vi "general data plot.vi"() -> ()   [LabVIEW 2021]
panel:
  in  "length":i32
  in  "start":i32
  out "min value":dbl
  out "max value":dbl=7.0
  in  "Data channel":u16(ring) items=["magitude", "phase", "i", "q"]
  in  "y bin":i32=100
  in  "x bin":i32=100
  in  "Tab Control":T1(tab)
  out "Curves":cluster{dbl[], dbl[]}[](graph)=[{[10.0, 20.0, 30.0, 40.0, 50.0, 60.0, 70.0, 80.0, 90.0, 100.0, 110.0, 120.0, 130.0, 140.0, 150.0, 160.0, 170.0, 180.0, 190.0, 200.0, 210.0, 220.0, 230.0, 240.0, 250.0, 260.0, 270.0, 280.0, 290.0, 300.0, 310.0, 320.0, 330.0, 340.0, 350.0, 360.0, 370.0, 380.0, 390.0, 400.0, 410.0, 420.0, 430.0, 440.0, 450.0, 460.0, 470.0, 480.0, 490.0, 500.0, 510.0, 520.0, 530.0, 540.0, 550.0, 560.0, 570.0, 580.0, 590.0, 600.0, 610.0, 620.0, 630.0, 640.0, 650.0, 660.0, 670.0, 680.0, 690.0, 700.0, 710.0, 720.0, 730.0, 740.0, 750.0, 760.0, 770.0, 780.0, 790.0, 800.0, 810.0, 820.0, 830.0, 840.0, 850.0, 860.0, 870.0, 880.0, 890.0, 900.0, 910.0, 920.0, 930.0, 940.0, 950.0, 960.0, 970.0, 980.0, 990.0, 1000.0, 1010.0, 1020.0, 1030.0, 1040.0, 1050.0, 1060.0, 1070.0, 1080.0, 1090.0, 1100.0, 1110.0, 1120.0, 1130.0, 1140.0, 1150.0, 1160.0, 1170.0, 1180.0, 1190.0, 1200.0, 1210.0, 1220.0, 1230.0, 1240.0, 1250.0, 1260.0, 1270.0, 1280.0, 1290.0, 1300.0, 1310.0, 1320.0, 1330.0, 1340.0, 1350.0, 1360.0, 1370.0, 1380.0, 1390.0, 1400.0, 1410.0, 1420.0, 1430.0, 1440.0, 1450.0, 1460.0, 1470.0, 1480.0, 1490.0, 1500.0, 1510.0, 1520.0, 1530.0, 1540.0, 1550.0, 1560.0, 1570.0, 1580.0, 1590.0, 1600.0, 1610.0, 1620.0, 1630.0, 1640.0, 1650.0, 1660.0, 1670.0, 1680.0, 1690.0, 1700.0, 1710.0, 1720.0, 1730.0, 1740.0, 1750.0, 1760.0, 1770.0, 1780.0, 1790.0, 1800.0, 1810.0, 1820.0, 1830.0, 1840.0, 1850.0, 1860.0, 1870.0, 1880.0, 1890.0, 1900.0, 1910.0, 1920.0, 1930.0, 1940.0, 1950.0, 1960.0, 1970.0, 1980.0, 1990.0, 2000.0, 2010.0, 2020.0, 2030.0, 2040.0, 2050.0, 2060.0, 2070.0, 2080.0, 2090.0, 2100.0, 2110.0, 2120.0, 2130.0, 2140.0, 2150.0, 2160.0, 2170.0, 2180.0, 2190.0, 2200.0, 2210.0, 2220.0, 2230.0, 2240.0, 2250.0, 2260.0, 2270.0, 2280.0, 2290.0, 2300.0, 2310.0, 2320.0, 2330.0, 2340.0, 2350.0, 2360.0, 2370.0, 2380.0, 2390.0, 2400.0, 2410.0, 2420.0, 2430.0, 2440.0, 2450.0, 2460.0, 2470.0, 2480.0, 2490.0, 2500.0, 2510.0, 2520.0, 2530.0, 2540.0, 2550.0, 2560.0, 2570.0, 2580.0, 2590.0, 2600.0, 2610.0, 2620.0, 2630.0, 2640.0, 2650.0, 2660.0, 2670.0, 2680.0, 2690.0, 2700.0, 2710.0, 2720.0, 2730.0, 2740.0, 2750.0, 2760.0, 2770.0, 2780.0, 2790.0, 2800.0, 2810.0, 2820.0, 2830.0, 2840.0, 2850.0, 2860.0, 2870.0, 2880.0, 2890.0, 2900.0, 2910.0, 2920.0, 2930.0, 2940.0, 2950.0, 2960.0, 2970.0, 2980.0, 2990.0], [0.00013367658539209515, 0.00012903053720947355, 0.00016939388297032565, 0.00011944288416998461, 0.00013280082202982157, 0.0001668874901952222, 0.0001486373512307182, 0.00016734786913730204, 0.00013047773973084986, 0.00011366923718014732, 0.00015346240252256393, 0.00014055744395591319, 0.00010855273285415024, 0.00014807406114414334, 9.691778541309759e-05, 0.0001037847250699997, 0.00015512084064539522, 0.00012899791181553155, 0.00010304365423507988, 0.00010984897380694747, 9.950714593287557e-05, 0.00012845687160734087, 9.946813952410594e-05, 0.00013071915600448847, 0.00010318124259356409, 7.330832886509597e-05, 9.540999599266797e-05, 8.451899338979274e-05, 0.00011770859418902546, 0.00010144653788302094, 0.00010661190026439726, 9.66657607932575e-05, 8.824256656225771e-05, 0.00011671280662994832, 0.0001153357297880575, 0.00012023511953884736, 0.00011908653686987236, 7.182291301432997e-05, 9.330980537924916e-05, 0.00012978495215065777, 0.00010747888882178813, 0.0001609536848263815, 0.00012383898138068616, 0.00012734768097288907, 0.00013171030150260776, 0.00016544826212339103, 0.00011794555030064657, 0.0001209946713061072, 0.00013883289648219943, 0.00011528369941515848, 0.00011119921691715717, 0.0001268050546059385, 0.0001389453827869147, 0.0001333432155661285, 0.0001442368666175753, 0.00013873385614715517, 0.00015191496640909463, 0.0001383038325002417, 0.00016562323435209692, 0.0001503702369518578, 0.00018218863988295197, 0.00015577522572129965, 0.00013113849854562432, 0.0001594854547875002, 0.0001855860318755731, 0.00019237845845054835, 0.00016393935948144644, 0.00012862142466474324, 0.00020546221639961004, 0.00017347501125186682, 0.00016879066242836416, 0.00018185762746725231, 0.00021324920817278326, 0.0001671143400017172, 0.00017139053670689464, 0.00019904927466996014, 0.00020881103409919888, 0.0001565761340316385, 0.00017052458133548498, 0.00014252751134335995, 0.00014181881851982325, 0.0001779100566636771, 0.00014105757873039693, 0.00018711318261921406, 0.00016824345220811665, 0.00015031950897537172, 0.0002022298431256786, 0.0001394925347995013, 0.00019517798500601202, 0.00016337772831320763, 0.00016140898515004665, 0.00015929783694446087, 0.00019489617261569947, 0.0001588258455740288, 0.00019977384363301098, 0.00012394576333463192, 0.00013413015403784811, 0.00019717543909791857, 0.00018152548000216484, 0.0001585373393027112, 0.00018475871183909476, 0.0001751347881508991, 0.00018880412972066551, 0.00014899946108926088, 0.00014845613623037934, 0.0001744086475810036, 0.0001450015843147412, 0.00016606866847723722, 0.00014761251804884523, 0.00012996570148970932, 0.000138217699714005, 0.00010744725295808166, 0.00014905130956321955, 0.00011166420881636441, 0.0001041400246322155, 0.0001146040522144176, 7.99687477410771e-05, 7.002366328379139e-05, 0.00017626908083911985, 0.00010617077350616455, 9.990988473873585e-05, 6.87278006807901e-05, 8.242046169470996e-05, 8.596655243309215e-05, 0.00014996137178968638, 8.169219654519111e-05, 0.0001243894948856905, 0.00014897635264787823, 0.0001250183704541996, 0.000117989067803137, 0.00012694876932073385, 0.00015508588694501668, 9.217203478328884e-05, 9.355860674986616e-05, 0.00010396670404588804, 9.367567690787837e-05, 8.306658128276467e-05, 9.193496953230351e-05, 9.813846554607153e-05, 0.00011742529750335962, 6.46550688543357e-05, 0.00013626340660266578, 0.00012126795627409592, 0.0001021269999910146, 0.0001304978650296107, 9.543891792418435e-05, 0.00013903676881454885, 0.00011544466542545706, 0.00013386114733293653, 0.0001186947338283062, 0.00010264376760460436, 0.00018659705528989434, 0.00010800208838190883, 0.00014367169933393598, 0.00011846152483485639, 7.385665958281606e-05, 0.0001364771305816248, 0.00011073373752878979, 0.00010194589413003996, 0.00014044092677067965, 8.428201545029879e-05, 0.00012676689948420972, 0.0001338515430688858, 0.00010269197809975594, 0.00023462837270926684, 0.00013209556345827878, 0.00010225973528577015, 0.000106790590507444, 0.00017195282271131873, 9.286184649681672e-05, 0.00012535882706288248, 0.000116468254418578, 9.88127212622203e-05, 0.00010617675434332341, 7.647919119335711e-05, 9.201795910485089e-05, 0.00010408402886241674, 9.458380372961983e-05, 0.0001077998531400226, 0.00011431352322688326, 0.00010332229430787265, 0.00011219579027965665, 0.0001334812113782391, 0.00014534480578731745, 0.00011573600932024419, 6.758727977285162e-05, 0.0001744368055369705, 0.00016830879030749202, 0.00017424295947421342, 0.00016627485456410795, 0.00012254131434019655, 9.647793922340497e-05, 7.145500421756878e-05, 0.0001961914385901764, 7.151101453928277e-05, 0.00012814125511795282, 9.786655573407188e-05, 0.00010398540325695649, 0.00010584685514913872, 0.00015125608479138464, 0.00012826750753447413, 5.975702151772566e-05, 0.00013089587446302176, 0.00012053469254169613, 0.00015860950225032866, 6.76583731546998e-05, 8.026184514164925e-05, 0.00013365043560042977, 6.834783562226221e-05, 5.882106052013114e-05, 7.937144255265594e-05, 8.463740959996358e-05, 8.238392183557153e-05, 9.121077164309099e-05, 0.00012566435907501727, 5.283867722027935e-05, 0.0001325753692071885, 0.0001193397692986764, 0.00011944347352255136, 0.00010491804277990013, 7.044597441563383e-05, 7.60913681006059e-05, 9.172792488243431e-05, 0.00011764467490138486, 5.072560816188343e-05, 5.034092100686394e-05, 9.650958236306906e-05, 0.00011145589814987034, 8.698977762833238e-05, 0.00013060042692814022, 7.508155249524862e-05, 4.039569466840476e-05, 0.00012688440619967878, 8.248807716881856e-05, 0.0001391138503095135, 0.00011811658623628318, 0.0001329777151113376, 0.0001297980488743633, 0.00011801200162153691, 7.027927495073527e-05, 8.611835073679686e-05, 8.903844718588516e-05, 5.4920932598179206e-05, 0.00010779354488477111, 8.671233081258833e-05, 7.775093399686739e-05, 0.00012373703066259623, 0.00010819485760293901, 0.00010179568198509514, 8.725826046429574e-05, 9.490929369349033e-05, 0.0001120992237702012, 0.0001260258286492899, 6.4598280005157e-05, 0.00011466383148217574, 0.00014919301611371338, 9.42891783779487e-05, 9.435992251383141e-05, 0.0001149402596638538, 8.329037518706173e-05, 0.00010850686521735042, 0.0001287714985664934, 0.00013188911543693393, 0.00011211052333237603, 0.0001296363479923457, 0.0001389684621244669, 0.0001123499168897979, 9.72454363363795e-05, 9.088624938158318e-05, 9.20691090868786e-05, 8.7498570792377e-05, 0.0001258686388609931, 0.00013619156379718333, 8.844014519127086e-05, 0.00012676880578510463, 8.672325202496722e-05, 0.00013719592243433, 0.000103384954854846, 7.913039007689804e-05, 7.551917224191129e-05, 7.993963663466275e-05, 0.0001514438772574067, 0.000121453391329851, 0.00014526258746627718, 0.00011735747830243781, 9.341667464468628e-05, 8.561307186027989e-05, 0.00013149157166481018, 0.00010279854177497327, 9.32314433157444e-05, 0.0001331145758740604, 8.938983228290454e-05, 0.00013474171282723546, 0.0001676843239692971, 8.821023220662028e-05, 0.00011201468441868201, 0.0001366356445942074, 0.00013054072041995823, 0.00016769583453424275]}]
  out "distribution":dbl[][](graph)
  in  "Dist Marker Values":cluster{"Numeric":dbl, "Color Box":u32}[](array[cluster])=[{"Numeric"=0.0, "Color Box"=16448250}, {"Numeric"=10.0, "Color Box"=16711686}, {"Numeric"=14.0, "Color Box"=16860}]
  out "Y Cut":T2(graph)
  out "Intensity plot":dbl[][](graph)
  in  "Intensity Marker Values":cluster{"Numeric":dbl, "Color Box":u32}[](array[cluster])
  out "error out":errorcluster
  out "Axis array":dbl[](array[numeric])
  in  "Y Label":string(combo)="Mag"
  in  "X Label":string(combo)="Length ns"
  in  "y col":i32=1
  in  "x col":i32
  in  "Plot Type":string(combo)="iq vs x"
  in  "Plot":bool
  out "Status":string(combo)="Idle"
  in  "Stop":bool
  in  "update":bool
  in  "Data files":i32[](listbox)=[168]
  in  "Main folder path":path=path "C:/Users/dvh-collab-user/Desktop/20230313 Robert sample"
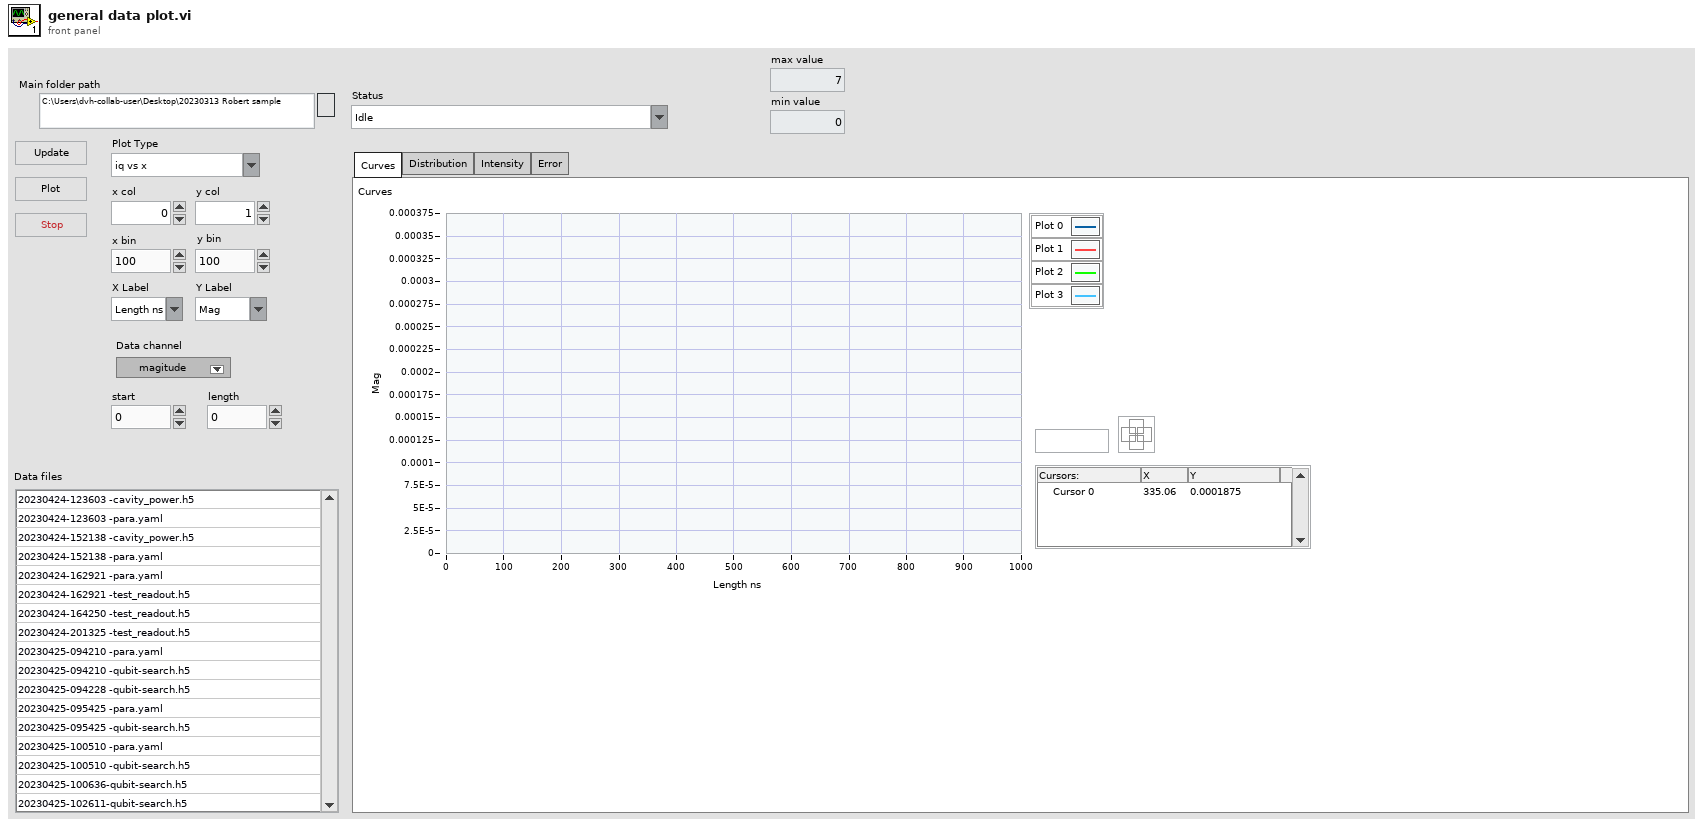
[diagram p1: front panel]
types:
  T1 = enum32{"Curves", "Distribution", "Intensity", "Error"}
  T2 = cluster{"Axis array":dbl[], "Intensity plot":dbl[]}
  T3 = cluster{" x min":dbl, "x step":dbl, "y min":dbl, "y step":dbl}
  T4 = cluster{"xname":string, "x_offset":dbl, "x_step":dbl, "yname":string, "y_offset":dbl, "y_step":dbl}
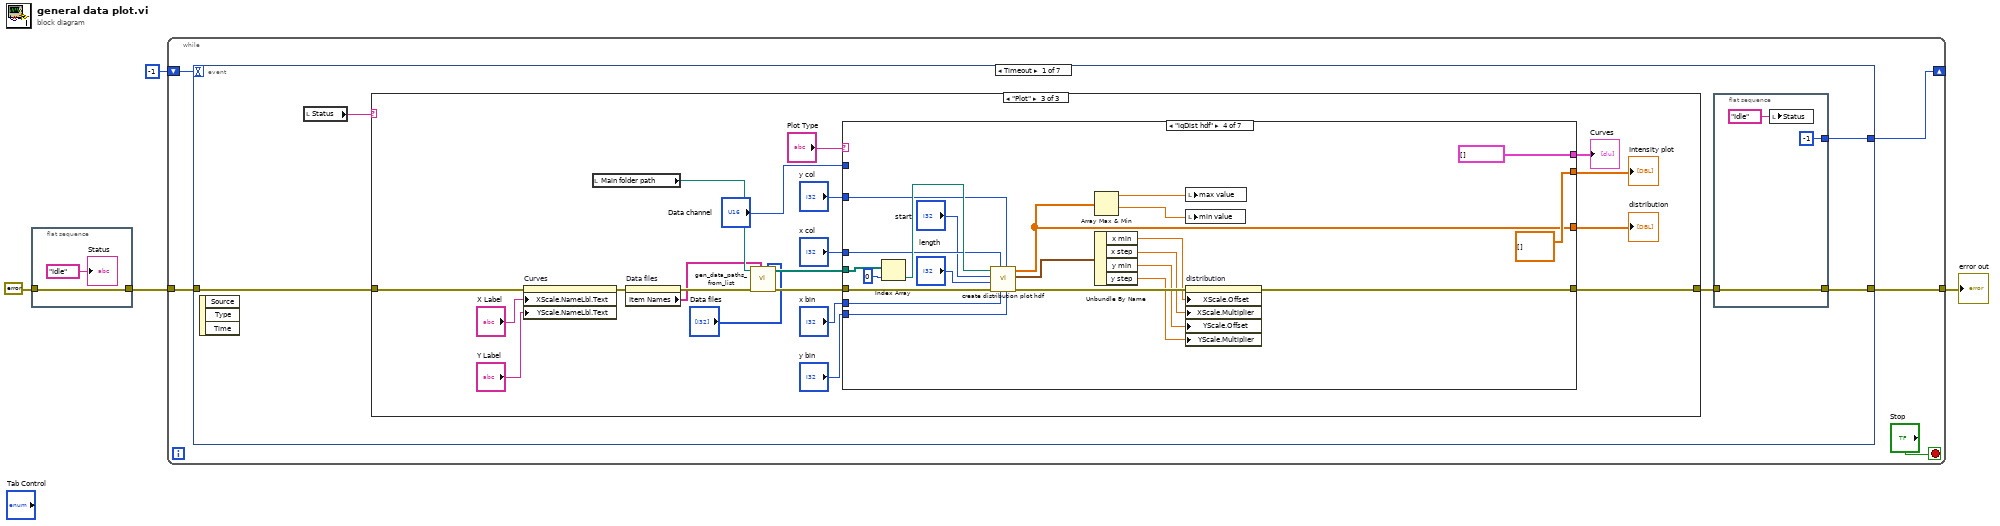
[diagram p0: block diagram]
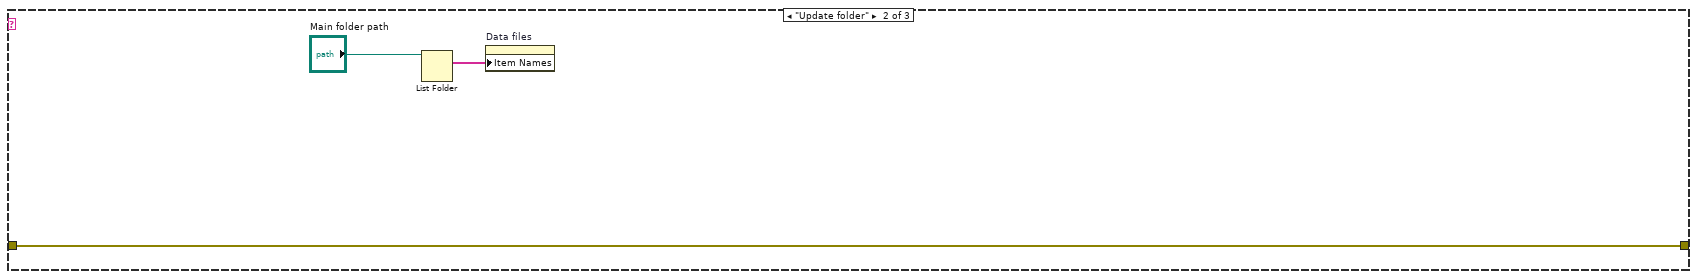
[diagram p3: hidden frame]
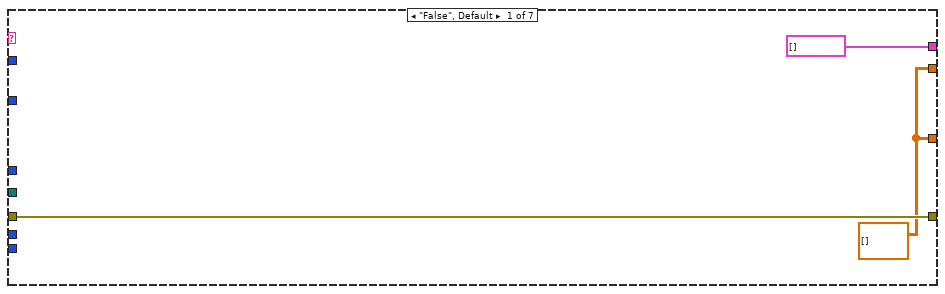
[diagram p4: hidden frame]
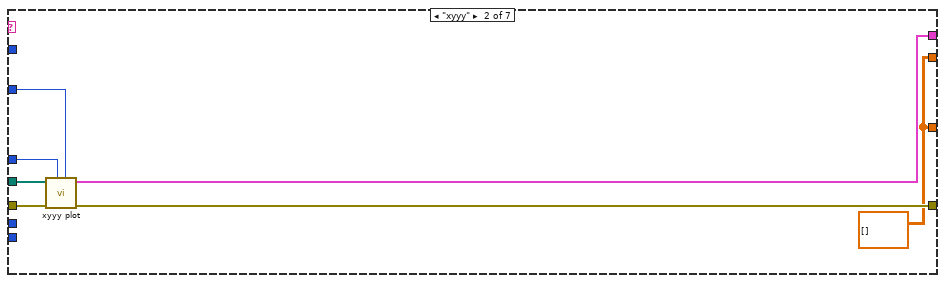
[diagram p5: hidden frame]
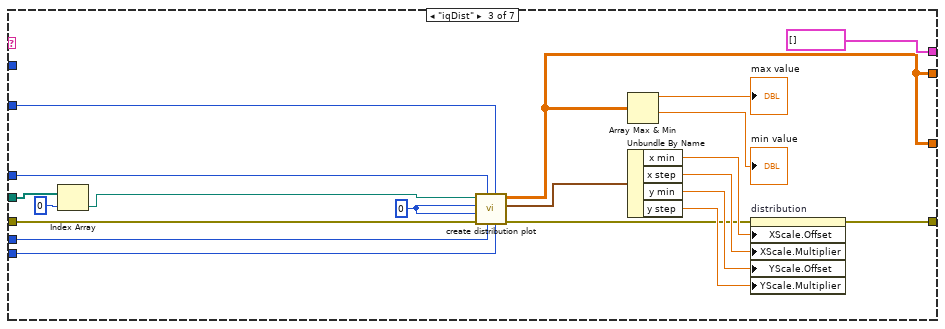
[diagram p6: hidden frame]
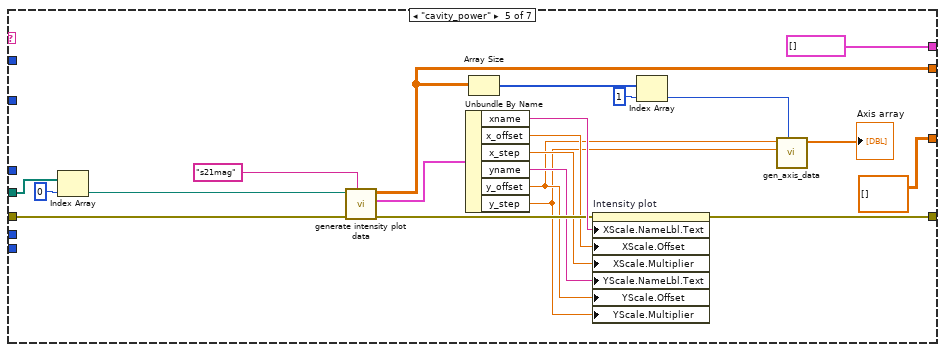
[diagram p7: hidden frame]
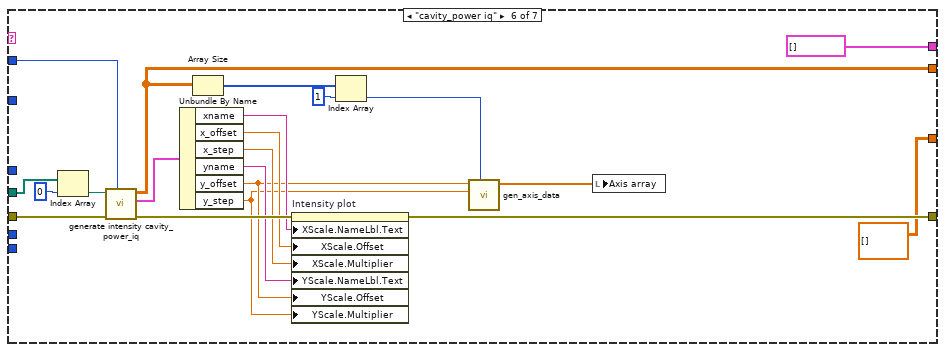
[diagram p8: hidden frame]
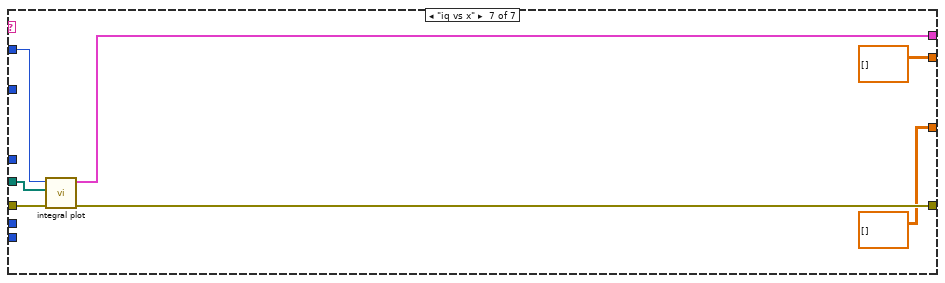
[diagram p9: hidden frame]
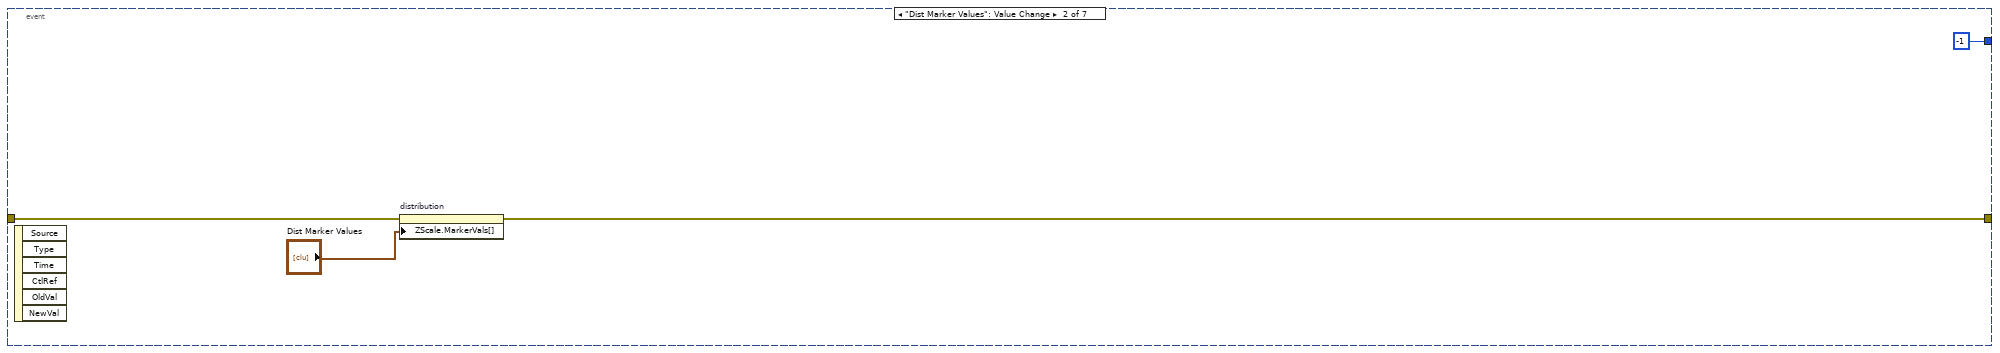
[diagram p10: hidden frame]
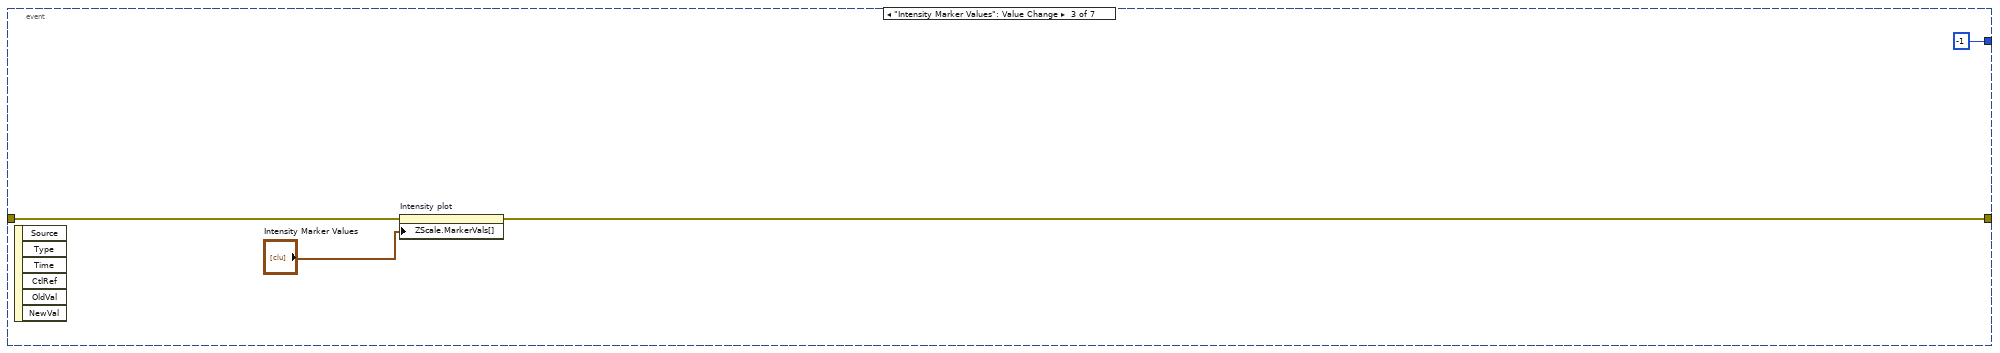
[diagram p11: hidden frame]
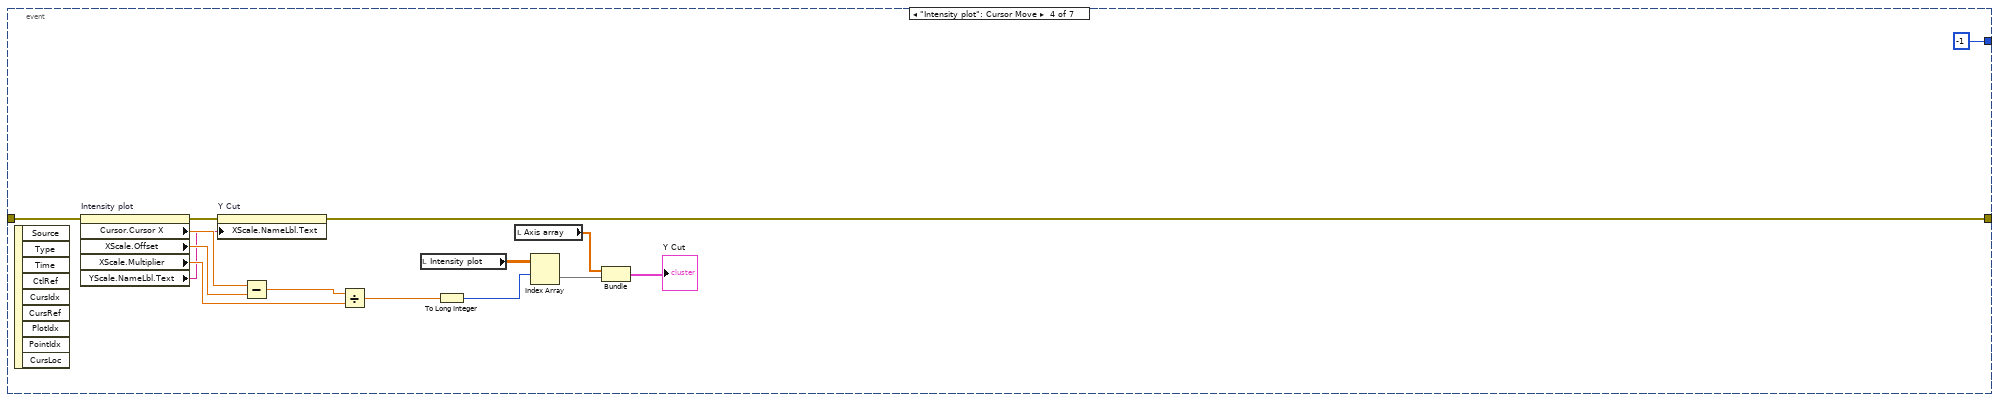
[diagram p12: hidden frame]
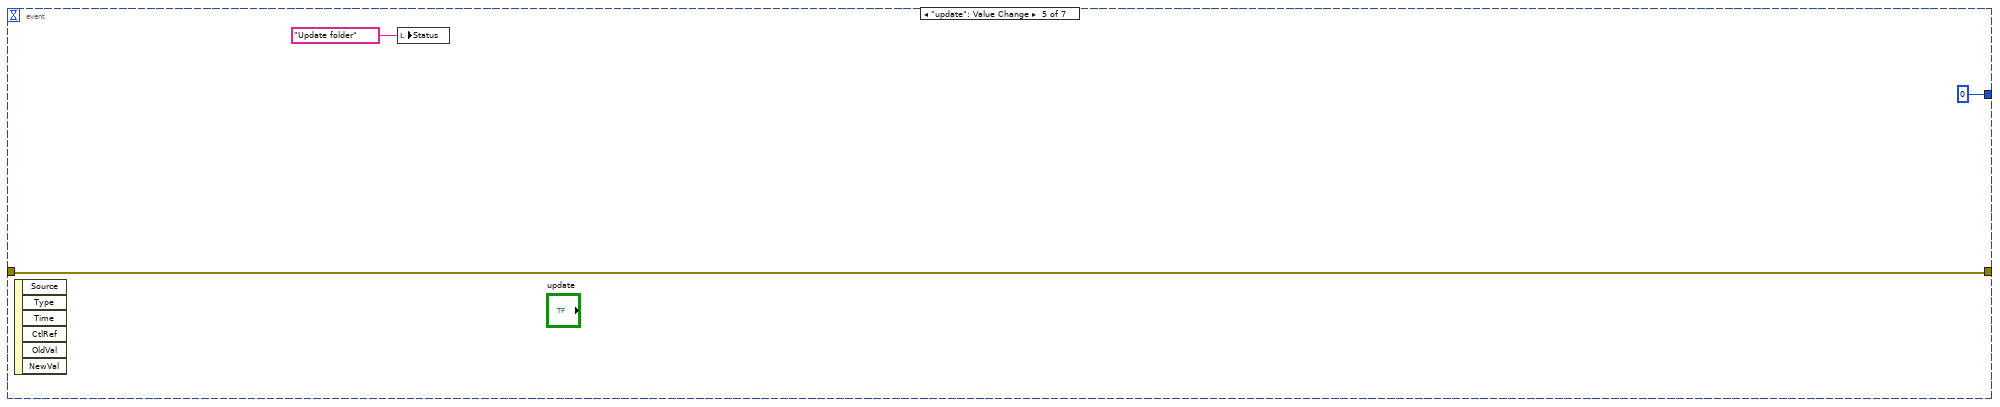
[diagram p13: hidden frame]
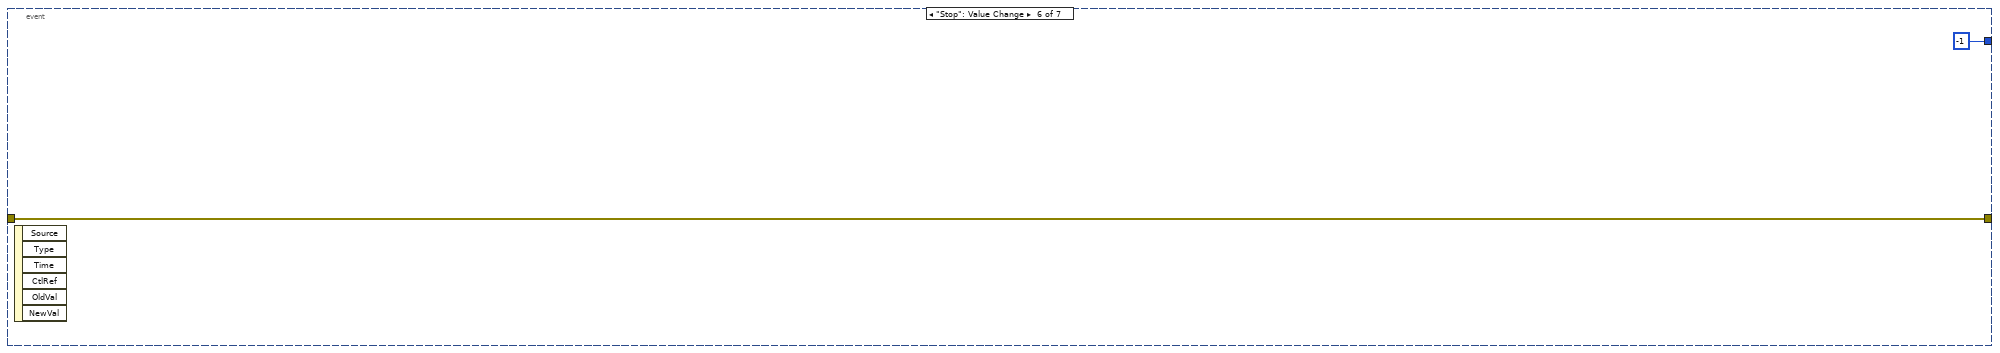
[diagram p14: hidden frame]
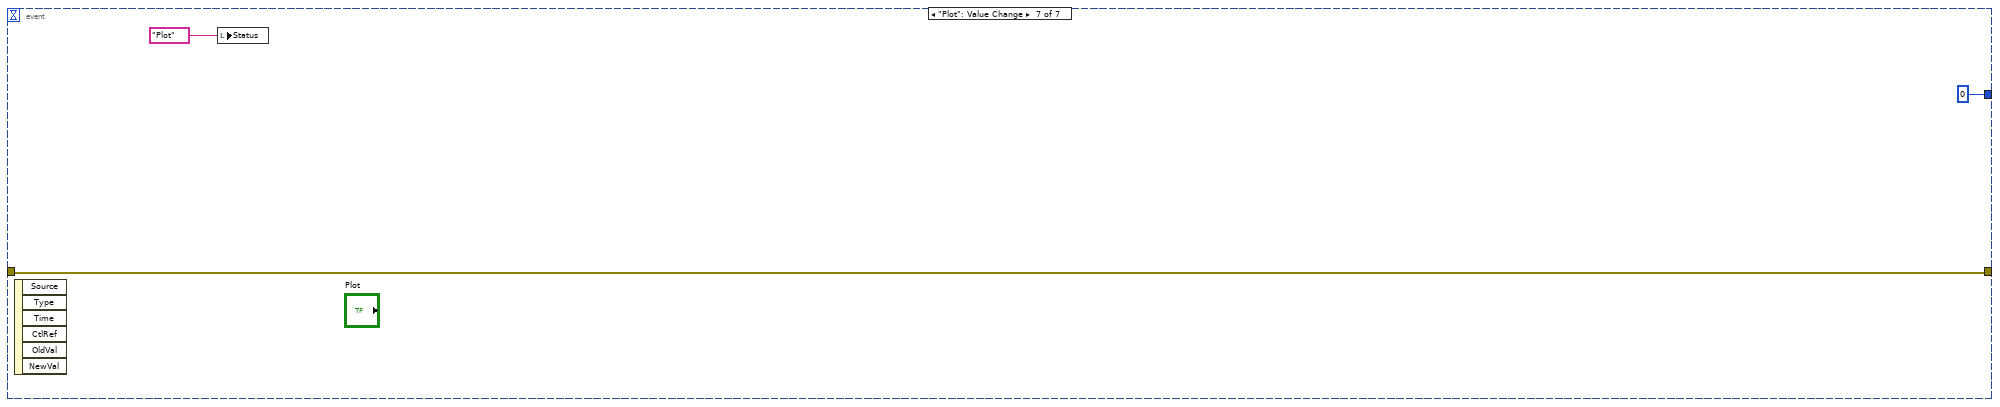
[diagram p15: hidden frame]
diagram:
  n1 = flat-sequence {
    tunnel: [w5] -> w2
    tunnel: errorcluster {"status"=FALSE, "code"=0, "source"=""} ("error in") -> [w5]
    frame #0 {
      "Status" <- "Idle" ("Status")
    }
  }
  n2 = while {
    shift-right: [w10] -> _
    shift-left: -1 -> [w11]
    tunnel: w2 -> [w9]
    tunnel: [w8] -> w1
    stop <- "Stop" stop-if-true
    n3 = event shown="[0] Timeout" {
      selector: _ -> [_ _ _ _ _ _ _]
      dyn-events: _ -> [_ _ _ _ _ _ _]
      timeout: w11 -> [_ _ _ _ _ _ _]
      tunnel: [w12 -1 -1 -1 0 -1 0] -> w10
      tunnel: w9 -> [w15 w147 w150 w167 w168 w172 w175]
      tunnel: [w13 w145 w152 w154 w168 w172 w175] -> w8
      event Timeout {
        n4 = event-data() -> ()  [unwired: 1 in, 3 out]
        n5 = local read "Status"() -> (w16:string)
        n6 = case shown="\"Plot\"" w16 {
          tunnel: [w20 w21 w39] -> w14
          tunnel: w15 -> [w20 w21 w32]
          frame "False", Default {
          }
          frame "Update folder" {
            n7 = List Folder(path="Main folder path") -> (filenames=w23:string[])  [unwired: 3 in, 3 out]
            n8 = property on="Data files" class="LstBox (strict)"("Item Names"=w23) -> ()  [unwired: 2 in, 2 out]
          }
          frame "Plot" {
            n9 = property on="Curves" class="XYGraph (strict)"(error in=w32, "XScale.NameLbl.Text"="X Label", "YScale.NameLbl.Text"="Y Label") -> (error out=w31:errorcluster)  [unwired: 1 in, 1 out]
            n10 = local read "Main folder path"() -> (w42:path)
            n11 = property on="Data files" class="LstBox (strict)"(error in=w31) -> (error out=w36:errorcluster, "Item Names"=w35:string[])  [unwired: 1 in, 1 out]
            n12 = call "gen_data_paths_from_list.vi"("Data index"="Data files", "Item Names"=w35, "error in (no error)"=w36, "Folder path"=w42) -> ("error out"=w40:errorcluster, "Array path"=w41:path[])  [unwired: 6 in]
            n13 = case shown="\"iqDist hdf\"" "Plot Type" {
              tunnel: w41 -> [_ w53 w72 w94 w114 w137 w141]
              tunnel: w40 -> [w45 w52 w69 w91 w111 w132 w144]
              tunnel: [w45 w51 w60 w92 w107 w130 w140] -> w39
              tunnel: [cluster{dbl[], dbl[]}[] [] ("output cluster") w50 cluster{dbl[], dbl[]}[] [] ("output cluster") cluster{dbl[], dbl[]}[] [] ("output cluster") cluster{dbl[], dbl[]}[] [] ("output cluster") cluster{dbl[], dbl[]}[] [] ("output cluster") w142] -> w38
              tunnel: "y col" -> [_ w49 w67 w87 _ _ _]
              tunnel: "x col" -> [_ w48 w68 w88 _ _ _]
              tunnel: [w44 w47 w57 w78 dbl[][] [] ("Intensity Graph") dbl[][] [] ("Intensity Graph") dbl[][] [] ("Intensity Graph")] -> w28
              tunnel: [w44 w47 w57 dbl[][] [] ("Data out") w101 w124 dbl[][] [] ("Data out")] -> w27
              tunnel: "x bin" -> [_ _ w59 w86 _ _ _]
              tunnel: "y bin" -> [_ _ w58 w85 _ _ _]
              tunnel: "Data channel" -> [_ _ _ _ _ w117 w143]
              frame "False", Default {
                w44 = dbl[][] [] ("Intensity Graph")
              }
              frame "xyyy" {
                w47 = dbl[][] [] ("Intensity Graph")
                n14 = call "xyyy plot.vi"("Y column"=w49, "X column"=w48, "error in (no error)"=w52, "file path (dialog if empty)"=w53) -> ("error out"=w51:errorcluster, "output cluster"=w50:cluster{dbl[], dbl[]}[])  [unwired: 6 in]
              }
              frame "iqDist" {
                w54 = 0 ("start")
                n15 = Index Array(array=w72, index=0) -> (element=w70:path)
                n16 = call "create distribution plot.vi"("y bin"=w58, "y row"=w67, "x bin"=w59, "x row"=w68, "error in (no error)"=w69, "length"=w54, "start"=w54, "Path"=w70) -> ("error out"=w61:errorcluster, "Cluster"=w66:T3, "Intensity Graph"=w57:dbl[][])  [unwired: 1 in]
                n17 = Array Max & Min(array=w57) -> (max value=→"max value":dbl, min value=→"min value":dbl)  [unwired: 2 out]
                n18 = Unbundle By Name(w66) -> ("x min"=w65:dbl, "x step"=w64:dbl, "y min"=w63:dbl, "y step"=w62:dbl)
                n19 = property on="distribution" class="IntGraph (strict)"(error in=w61, "XScale.Offset"=w65, "XScale.Multiplier"=w64, "YScale.Offset"=w63, "YScale.Multiplier"=w62) -> (error out=w60:errorcluster)  [unwired: 1 in, 1 out]
              }
              frame "iqDist hdf" {
                n20 = Index Array(array=w94, index=0) -> (element=w89:path)
                n21 = call "create distribution plot hdf.vi"("y bin"=w85, "y row"=w87, "x bin"=w86, "x row"=w88, "error in (no error)"=w91, "length"="length", "start"="start", "Path"=w89) -> ("error out"=w90:errorcluster, "Cluster"=w84:T3, "Intensity Graph"=w78:dbl[][])  [unwired: 1 in]
                n22 = Array Max & Min(array=w78) -> (max value=w77:dbl, min value=w76:dbl)  [unwired: 2 out]
                n23 = Unbundle By Name(w84) -> ("x min"=w83:dbl, "x step"=w82:dbl, "y min"=w81:dbl, "y step"=w80:dbl)
                n24 = local write "max value"(w77) -> ()
                n25 = local write "min value"(w76) -> ()
                n26 = property on="distribution" class="IntGraph (strict)"(error in=w90, "XScale.Offset"=w83, "XScale.Multiplier"=w82, "YScale.Offset"=w81, "YScale.Multiplier"=w80) -> (error out=w92:errorcluster)  [unwired: 1 in, 1 out]
              }
              frame "cavity_power" {
                n27 = Index Array(array=w114, index=0) -> (element=w113:path)
                n28 = call "generate intensity plot data.vi"("Dataset Path"="s21mag", "error in (no error)"=w111, "path"=w113) -> ("error out"=w108:errorcluster, "Attribute Value(s) out"=w110:T4, "Data out"=w101:dbl[][])  [unwired: 6 in]
                n29 = Unbundle By Name(w110) -> ("xname"=w109:string, "x_offset"=w106:dbl, "x_step"=w105:dbl, "yname"=w104:string, "y_offset"=w103:dbl, "y_step"=w102:dbl)
                n30 = Array Size(array=w101) -> (size(s)=w100:i32[])
                n31 = property on="Intensity plot" class="IntGraph (strict)"(error in=w108, "XScale.NameLbl.Text"=w109, "XScale.Offset"=w106, "XScale.Multiplier"=w105, "YScale.NameLbl.Text"=w104, "YScale.Offset"=w103, "YScale.Multiplier"=w102) -> (error out=w107:errorcluster)  [unwired: 1 in, 1 out]
                n32 = Index Array(array=w100, index=1) -> (element=w98:i32)
                n33 = call "gen_axis_data.vi"("size"=w98, "step"=w102, "start"=w103) -> ("Array"=→"Axis array":dbl[])  [unwired: 8 in]
              }
              frame "cavity_power iq" {
                n34 = Index Array(array=w137, index=0) -> (element=w135:path)
                n35 = call "generate intensity cavity_power_iq.vi"("Data channel"=w117, "error in (no error)"=w132, "path"=w135) -> ("error out"=w131:errorcluster, "Attribute Value(s) out"=w129:T4, "Data out"=w124:dbl[][])  [unwired: 6 in]
                n36 = Unbundle By Name(w129) -> ("xname"=w128:string, "x_offset"=w127:dbl, "x_step"=w126:dbl, "yname"=w125:string, "y_offset"=w122:dbl, "y_step"=w121:dbl)
                n37 = Array Size(array=w124) -> (size(s)=w134:i32[])
                n38 = property on="Intensity plot" class="IntGraph (strict)"(error in=w131, "XScale.NameLbl.Text"=w128, "XScale.Offset"=w127, "XScale.Multiplier"=w126, "YScale.NameLbl.Text"=w125, "YScale.Offset"=w122, "YScale.Multiplier"=w121) -> (error out=w130:errorcluster)  [unwired: 1 in, 1 out]
                n39 = Index Array(array=w134, index=1) -> (element=w123:i32)
                n40 = call "gen_axis_data.vi"("size"=w123, "step"=w121, "start"=w122) -> ("Array"=w120:dbl[])  [unwired: 8 in]
                n41 = local write "Axis array"(w120) -> ()
              }
              frame "iq vs x" {
                n42 = call "integral plot.vi"("error in (no error)"=w144, "Array path"=w141, "Data channel"=w143) -> ("error out"=w140:errorcluster, "Array"=w142:cluster{"Data out":dbl[], "Data out":dbl[]}[])  [unwired: 7 in]
              }
            }
            "Curves" <- w38
            "distribution" <- w28
            "Intensity plot" <- w27
          }
        }
        n43 = flat-sequence {
          tunnel: [w18] -> w13
          tunnel: w14 -> [w18]
          tunnel: [-1] -> w12
          frame #0 {
            n44 = local write "Status"("Idle" ("Status")) -> ()
          }
        }
      }
      event "Dist Marker Values": Value Change {
        n45 = event-data() -> ()  [unwired: 1 in, 6 out]
        n46 = property on="distribution" class="IntGraph (strict)"(error in=w147, "ZScale.MarkerVals[]"="Dist Marker Values") -> (error out=w145:errorcluster)  [unwired: 1 in, 1 out]
      }
      event "Intensity Marker Values": Value Change {
        n47 = event-data() -> ()  [unwired: 1 in, 6 out]
        n48 = property on="Intensity plot" class="IntGraph (strict)"(error in=w150, "ZScale.MarkerVals[]"="Intensity Marker Values") -> (error out=w152:errorcluster)  [unwired: 1 in, 1 out]
      }
      event "Intensity plot": Cursor Move {
        n49 = event-data() -> ()  [unwired: 1 in, 9 out]
        n50 = property on="Intensity plot" class="IntGraph (strict)"(error in=w167) -> (error out=w156:errorcluster, "Cursor.Cursor X"=w161:dbl, "XScale.Offset"=w160:dbl, "XScale.Multiplier"=w158:dbl, "YScale.NameLbl.Text"=w155:string)  [unwired: 1 in, 1 out]
        n51 = property on="Y Cut" class="XYGraph (strict)"(error in=w156, "XScale.NameLbl.Text"=w155) -> (error out=w154:errorcluster)  [unwired: 1 in, 1 out]
        n52 = Subtract(x=w161, y=w160) -> (x-y=w159:dbl)
        n53 = Divide(x=w159, y=w158) -> (x/y=w157:dbl)
        n54 = local read "Intensity plot"() -> (w166:dbl[][])
        n55 = To Long Integer(number=w157) -> (32bit integer=w165:i32)
        n56 = local read "Axis array"() -> (w164:dbl[])
        n57 = Index Array(array=w166, index (row)=w165) -> (element=w163:dbl[])  [unwired: 1 in]
        n58 = Bundle("Axis array"=w164, "Intensity plot"=w163) -> (→"Y Cut":T2)  [unwired: 1 in]
      }
      event "update": Value Change {
        n59 = event-data() -> ()  [unwired: 1 in, 6 out]
        n60 = local write "Status"("Update folder" ("Status")) -> ()
      }
      event "Stop": Value Change {
        n61 = event-data() -> ()  [unwired: 1 in, 6 out]
      }
      event "Plot": Value Change {
        n62 = event-data() -> ()  [unwired: 1 in, 6 out]
        n63 = local write "Status"("Plot" ("Status")) -> ()
      }
    }
  }
  "error out" <- w1
